vi "Dashboard Main.vi"() -> ()   [LabVIEW 2014]
uses:
  <vilib>/event_ctls.llb/eventvkey.ctl
  <vilib>/Rock Robotics/WPI/Dashboard/WPI_DashboardLogging Global.vi
  <vilib>/Rock Robotics/Network Tables/SD Read Numeric Array.vi
  <vilib>/Rock Robotics/Network Tables/SD Read Number.vi
  <vilib>/Rock Robotics/Network Tables/SD Write Number.vi
  <vilib>/Rock Robotics/Network Tables/SD Read Boolean.vi
  <vilib>/Utility/config.llb/Write Key (String).vi
  <vilib>/Utility/config.llb/Write Key (I32).vi
  <vilib>/Utility/config.llb/NI_LVConfig.lvlib
  <vilib>/Rock Robotics/Network Tables/SD Write String Array.vi
  <vilib>/Rock Robotics/Network Tables/SD Read String Array.vi
panel:
  out "Boolean":bool
  in  "Close Dashboard":bool
  in  "TCP":refnum<k5>
  in  "Rec Mode":enum32{"Stop", "Record", "Playback"}(radio)
  in  "Vision":u16(ring)=3 items=["Camera Off", "USB Camera SW", "USB Camera HW", "IP Camera"]
  out "Image Message":string="Timeout in Camera Communications"
  in  "Dashboard Tab":T1(tab)
  out "Current":dbl[](graph)
  out "Mutton Tank":dbl(knob) scale=0.0..6.0
  in  "AutoMode":enum16{"", "Straight", "Diagonal", "U-Turn"}(ring)
  in  "Camera Settings":T2={"Frame Rate"=30, "Compression"=30, "Size"=1} {"Frame Rate" scale=1.0..30.0; "Size" items=["640x480", "320x240", "160x120"]}
  out "Mode":T3(ring)=enum."Auto Disabled"
  in  "DB Camera Config":bool
  out "fps":dbl format="%#.1g"
  out "Mbps":dbl format="%#.1g"
  out "Mbps 2":bool
  out "Left Pwr":cluster{dbl, dbl}(slide)={0.0, -15.348837209302326} scale=-100.0..100.0
  out "Right Pwr":cluster{dbl, dbl}(slide)={0.0, -15.348837209302326} scale=-100.0..100.0
  out "Right Spd":dbl(slide) scale=-20.0..20.0
  out "Left Spd":dbl(slide) scale=-20.0..20.0
  out "High Gear?":bool
  in  "DB/String 9":string
  in  "DB/String 8":string
  in  "DB/String 7":string
  in  "DB/String 6":string
  in  "DB/String 5":string
  in  "DB/String 4":string
  in  "DB/String 3":string
  in  "DB/String 2":string
  in  "DB/String 1":string
  in  "DB/String 0":string
  in  "DB/Slider 0":dbl(slide) scale=0.0..5.0
  in  "DB/Slider 1":dbl(slide) scale=0.0..5.0
  in  "DB/Slider 2":dbl(slide) scale=0.0..5.0
  in  "DB/Slider 3":dbl(slide) scale=0.0..5.0
  out "DB/LED 3":bool
  out "DB/LED 2":bool
  out "DB/LED 1":bool
  out "DB/LED 0":bool
  in  "DB/Button 3":bool
  in  "DB/Button 2":bool
  in  "DB/Button 1":bool
  in  "DB/Button 0":bool caption="New Name"
  in  "Test Slider":dbl(slide) scale=0.0..100.0 scale format="%#_3g"
  in  "On/Off":bool caption="Solenoid"
  in  "Test Name":u16(ring) items=["Select the test to run...", "Example Test", "-------------------------------", "List of tests is built in robot code.", "Replace with your own automated tests."]
  in  "Test Tree":string(tree)
  in  "Motor":cluster{"Value":dbl, "Enable":bool} {"Value" scale=-1.0..1.0 scale format="%#_3g"}
  out "Progress":T4 {"Test Progress" scale=0.0..100.0}
  in  "Rev/Fwd":cluster{"Forward":bool, "Reverse":bool}
  in  "Test Ring":u16(ring) items=["Monochrome", "Color"]
  in  "Listbox":i32(listbox)
  out "Tree":string(tree)
  in  "Variables":string[](array[string])
  out "Camera Image":T5(plugin-control)
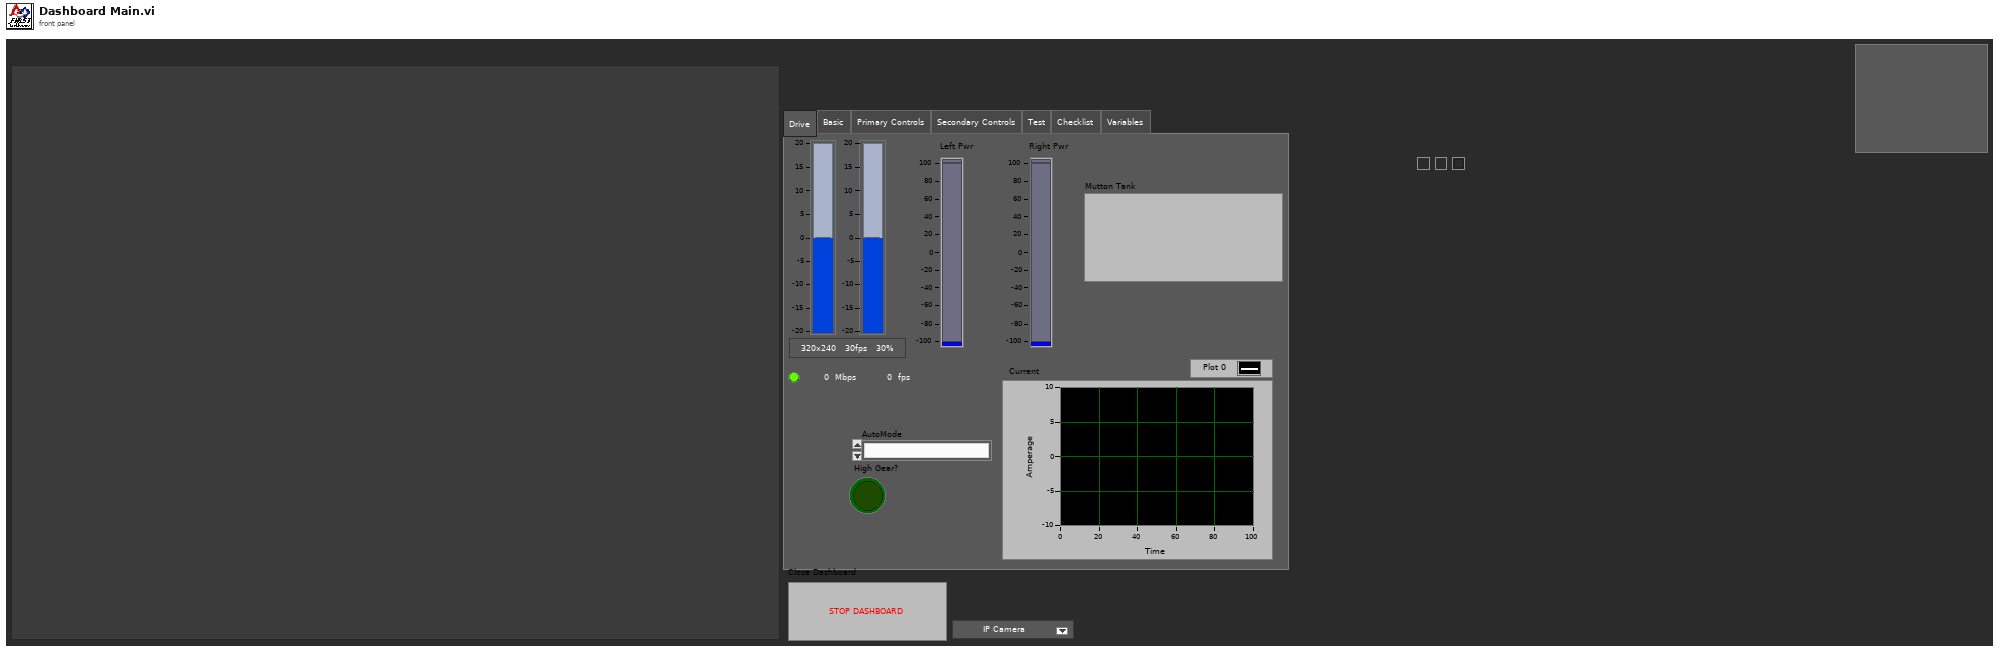
[diagram p1: front panel]
types:
  T1 = enum32{"Drive", "Basic", "Primary Controls", "Secondary Controls", "Test", "Checklist", "Variables"}
  T2 = cluster{"Frame Rate":i32, "Compression":i32, "Size":u16}
  T3 = enum8{"Tele-Op Disabled", "Tele-Op Enabled", "Auto Disabled", "Auto Enabled", "Test Disabled", "Test Enabled", "Disconnected", "No Code", "E-Stop"}
  T4 = cluster{"Test Progress":u8, "Test Progress Text":string}
  T5 = typedef "IMAQ Image.ctl" = refnum<image>
  T6 = enum32{"Drive", "Basic", "Custom", "Test", "Checklist", "Variables"}
  T7 = typedef "Image Type" = u32
  T8 = cluster{"Error Strings":string, "Disable Counts":cluster{u16, u16}, "Rail Faults":cluster{u16, u16, u16}, "Robot IP":string, "DB Mode":u8, "Event Info":cluster{"Name":string, "Type":u8, "Number":u16, "Replay":u8}, "Camera Addr":string}
  T9 = cluster{"Storage":cluster{"Disk Free":u64, "RAM Block":u32, "RAM free":u32}, "CPU Utilization":cluster{"CPU % ISR":sgl, "CPU % Time Crit":sgl, "CPU % Timed Str":sgl, "CPU % High":sgl, "CPU % Above":sgl, "CPU % Normal":sgl, "CPU % Low":sgl}, "CAN":cluster{"% Bus Utilization":sgl, "Bus Off Cnt":u32, "TX_FIFO Full Cnt":u32, "Receive Error Cnt":u8, "Transmit Error Cnt":u8}, "HID":cluster{"HID Outputs":u32, "Rumble Low":u16, "Rumble High":u16}[]}
  T10 = cluster{"Status bits":cluster{"Test Mode":bool, "Autonomous":bool, "Enabled":bool, "Code Start":bool, "Brownout":bool, "Reserved 2":bool, "Reserved 3":bool, "E-Stop":bool}, "Code Trace":cluster{"Disabled":bool, "TeleOp":bool, "Auto":bool, "Test":bool}, "Controller Type":enum16{"unknown", "cRIO", "roboRio"}, "Code?":enum16{"unknown", "noCode", "code"}, "Battery V":dbl}
  T11 = cluster{"Control Bits":cluster{"TestMode":bool, "Autonomous":bool, "Enabled":bool, "FMS Present":bool, bool, bool, bool, "E-Stop":bool}, "Team Station ":u8, "Countdown":sgl, "Joystick Values":cluster{"Axes":dbl[], "Buttons":bool[], "POVs":i16[]}[]}
  T12 = cluster{"Camera Image":refnum<vi>, "Dashboard Tab":refnum<vi>, "Boolean":refnum<vi>, "Vision":refnum<vi>, "Rec Mode":refnum<vi>, "Test Slider":refnum<vi>, "On/Off ":refnum<vi>, "Test Ring":refnum<vi>, "Rev/Fwd":refnum<vi>, "Test Name":refnum<vi>, "Motor":refnum<vi>, "Progress":refnum<vi>, "CheckList":refnum<vi>, "Tree":refnum<vi>, "Test Tree":refnum<vi>}
  T13 = typedef "NI_LVConfig.lvlib/Config Data RefNum.ctl" = refnum<k1>
  T14 = cluster{"Operation":enum16{"Update", "Clear"}, "Color Box":u32}[]
  T15 = typedef "eventvkey.ctl" = enum16{"ASCII", "Enter", "Return", "Shift", "Ctrl", "Alt", "Cmd", "Opt", "Caps", "NumLock", "Clear", "Break", "Up", "Down", "Left", "Right", "Insert", "Delete", "Home", "End", "PageUp", "PageDown", "Escape", "Help", "Pause", "ScrollLock", "F1", "F2", "F3", "F4", "F5", "F6", "F7", "F8", "F9", "F10", "F11", "F12", "F13", "F14", "F15", "F16", "F17", "F18", "F19", "F20", "F21", "F22", "F23", "F24", "Play", "VolumeUp", "VolumeDown", "Mute", "Two Byte Char"}
  T16 = cluster{"Image Size":bool, "Image Type":bool, "Pixel Value":bool, "ROI Information":bool, "Zoom Factor":bool}
  T17 = enum8{"Enabled", "Disabled", "Disabled and Grayed Out"}
  T18 = cluster{"Operation":enum16{"Update", "Clear"}, "Color Box":u32}
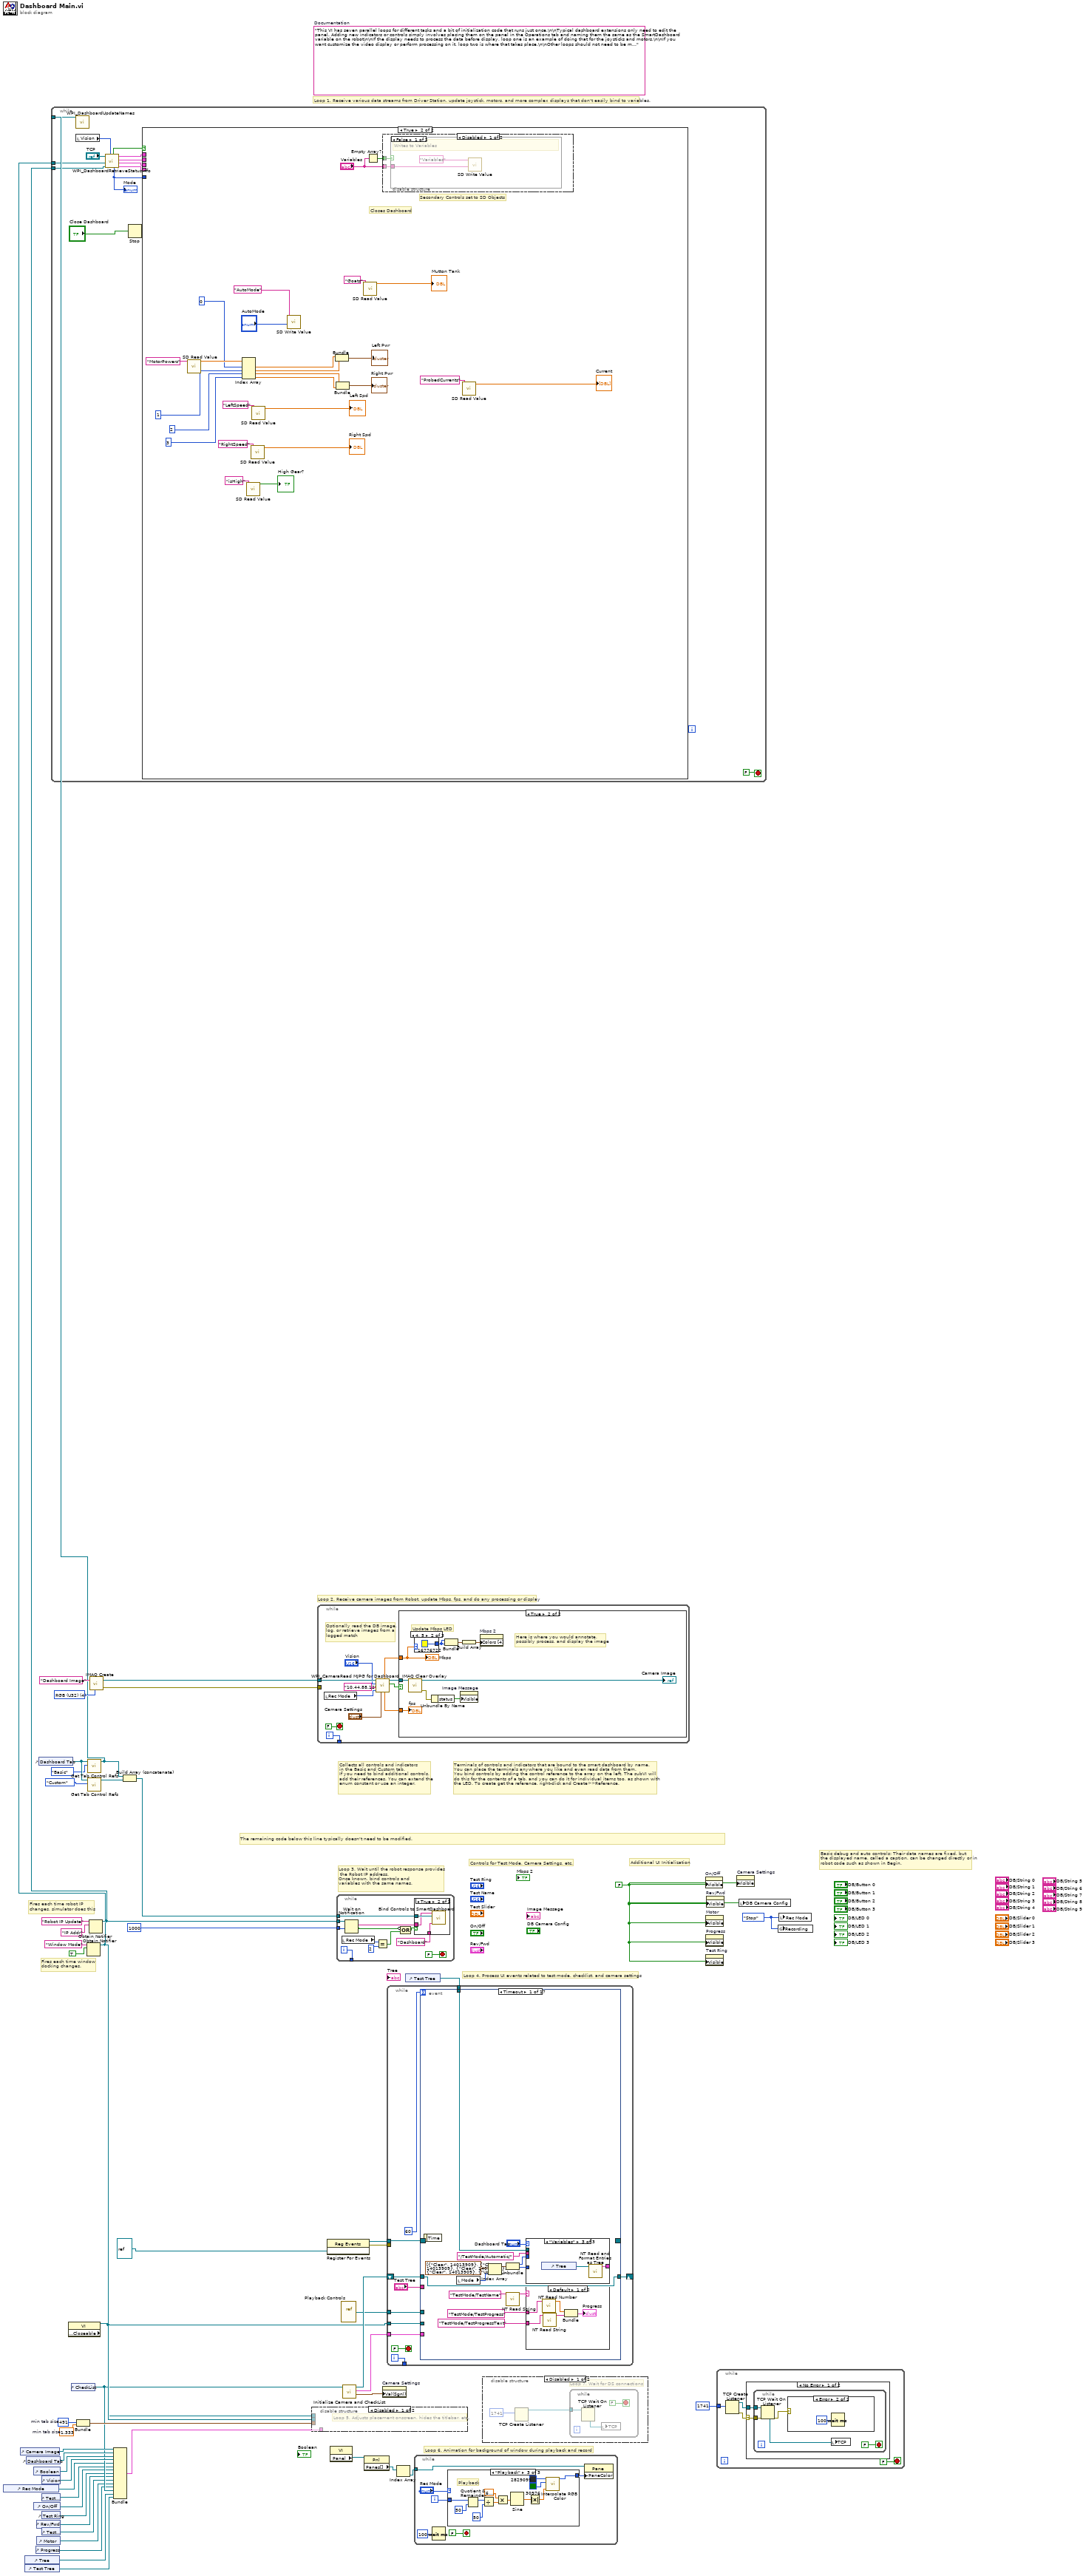
[diagram p0: block diagram]
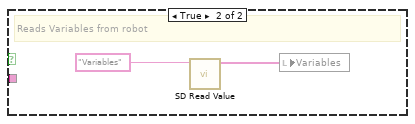
[diagram p7: hidden frame]
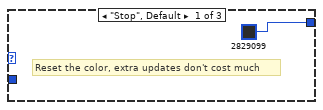
[diagram p9: hidden frame]
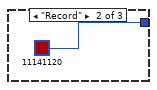
[diagram p10: hidden frame]
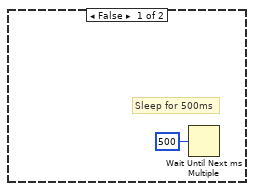
[diagram p12: hidden frame]
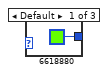
[diagram p13: hidden frame]
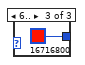
[diagram p14: hidden frame]
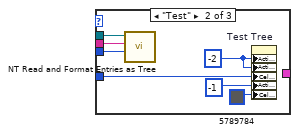
[diagram p16: hidden frame]
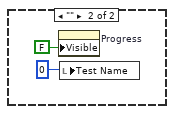
[diagram p17: hidden frame]
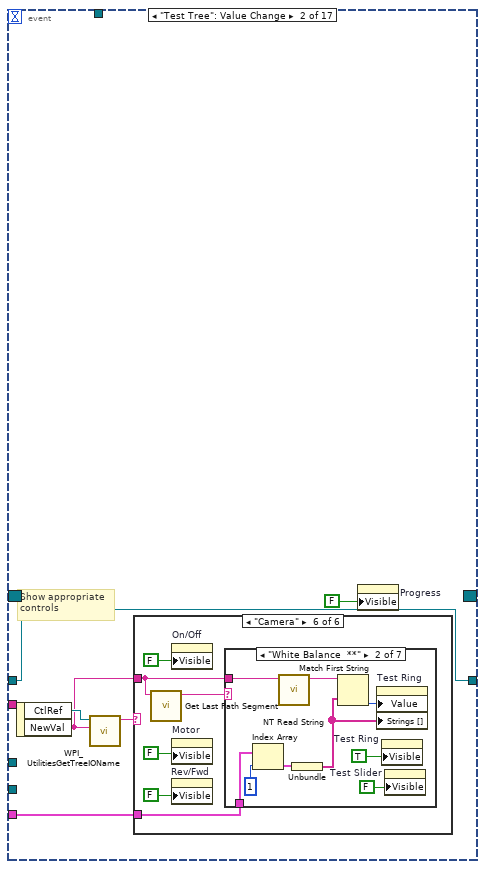
[diagram p18: hidden frame]
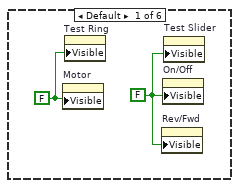
[diagram p19: hidden frame]
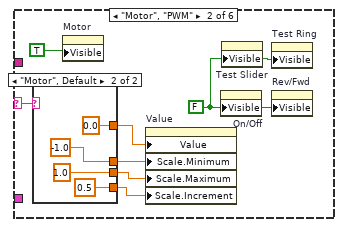
[diagram p20: hidden frame]
diagram:
  w23 = 491  # min tab size
  w22 = 1.333  # min tab size
  w31 = enum32{"Stop", "Record", "Playback"}."Stop" ("Rec Mode")
  w5 = FALSE ("Visible")
  (unwired) "This VI has seven parallel loops for different tasks and a bit of initialization code that runs just once.\n\nTypical dashboard extensions only need to edit the panel. Adding new indicators or controls simply involves placing them on the panel in the Operations tab and naming them the same as the SmartDashboard variable on the robot\n\nIf the display needs to process the data before display, loop one is an example of doing that for the joysticks and motors.\n\nIf you want customize the video display or perform processing on it, loop two is where that takes place.\n\nOther loops should not need to be modified. They are pretty standard, and document the task they perform."  # Documentation
  w51 = T7 4 items=["Grayscale (U8)", "Grayscale (I16)", "Grayscale (SGL)", "Complex (CSG)", "RGB (U32)", "HSL (U32)", "RGB (U64)"] ("Image Type")
  # "Basic debug and auto controls: Their data names are fixed, but\nthe displayed name, called a caption, can be changed directly or in\nrobot code such as shown in Begin."
  # "Controls for Test Mode, Camera Settings, etc."
  # "Additional UI Initialization"
  # "Loop 6. Animation for background of window during playback and record"
  # "Fires each time robot IP\nchanges, simulator does this"
  # "Fires each time window\ndocking changes."
  # "Collects all controls and indicators\nin the Basic and Custom tab.\nIf you need to bind additional controls,\nadd their references. You can extend the\nenum constant or use an integer."
  # "The remaining code below this line typically doesn't need to be modified."
  # "Loop 4. Process UI events related to test mode, checklist, and camera settings"
  # "Terminals of controls and indicators that are bound to the smart dashboard by name.\nYou can place the terminals anywhere you like and even read data from them.\nYou bind controls by adding the control reference to the array on the left. The subVI will\ndo this for the contents of a tab, and you can do it for individual items too, as shown with\nthe LED. To create get the reference, right-click and Create>>Reference."
  # "Loop 3. Wait until the robot response provides\n the Robot IP address.\nOnce known, bind controls and\nvariables with the same names."
  # "Loop 1. Receive various data streams from Driver Station, update joystick, motors, and more complex displays that don't easily bind to variables."
  # "Loop 2. Receive camera images from Robot, update Mbps, fps, and do any processing or display"
  n1 = control-ref of="Rec Mode"() -> (w11:refnum<vi>)
  n2 = control-ref of="Camera Image"() -> (w26:refnum<vi>)
  n3 = control-ref of="Tree"() -> (w15:refnum<vi>)
  n4 = control-ref of="Test Tree"() -> (w14:refnum<vi>)
  n5 = control-ref of="Dashboard Tab"() -> (w25:refnum<vi>)
  n6 = control-ref of="Boolean"() -> (w20:refnum<vi>)
  n7 = control-ref of="On/Off"() -> (w9:refnum<vi>)
  n8 = control-ref of="Progress"() -> (w6:refnum<vi>)
  n9 = control-ref of="Rev/Fwd"() -> (w7:refnum<vi>)
  n10 = control-ref of="Motor"() -> (w12:refnum<vi>)
  n11 = control-ref of="Dashboard Tab"() -> (w29:refnum<vi>)
  n12 = control-ref of="Test Slider"() -> (w10:refnum<vi>)
  n13 = control-ref of="Vision"() -> (w24:refnum<vi>)
  n14 = control-ref of="Test Ring"() -> (w8:refnum<vi>)
  n15 = control-ref of="Test Name"() -> (w13:refnum<vi>)
  n16 = property class="VI" props=["Front Panel.Closeable"]() -> (reference out=w30:refnum<vi>)  [unwired: 2 in, 2 out]
  n17 = control-ref of="CheckList"() -> (w16:refnum<vi>)
  n18 = Bundle("min tab size"=w23, "min tab size"=w22) -> (w21:cluster{"min tab size":i32, "min tab size":dbl})  [unwired: 1 in]
  n19 = Obtain Notifier(name (unnamed)="Window Mode", notification data type=TRUE) -> (notifier out=w2:refnum<notifier>)  [unwired: 2 in, 2 out]
  n20 = call <vilib>:"Get Tab Control Refs.vi"("Page Index"=T6."Basic" ("Dashboard Tab"), "TabControl in"=w29) -> ("ControlsOnPage"=w3:refnum<vi>[])  [unwired: 9 in]
  n21 = call <vilib>:"Get Tab Control Refs.vi"("Page Index"=T6."Custom" ("Dashboard Tab"), "TabControl in"=w29) -> ("ControlsOnPage"=w28:refnum<vi>[])  [unwired: 9 in]
  n22 = Obtain Notifier(name (unnamed)="Robot IP Update", notification data type="IP Addr" ("name (unnamed)")) -> (notifier out=w4:refnum<notifier>)  [unwired: 2 in, 2 out]
  n23 = while {
    tunnel: w4 -> [w59]
    tunnel: w3 -> [w58]
    tunnel: w2 -> [w54]
    stop <- FALSE stop-if-true
    n24 = call <vilib>:"WPI_DashboardUpdateNames.vi"("Controls on Tab"=w58) -> ()  [unwired: 11 in]
    n25 = local read "Vision"() -> (w56:u16)
    n26 = call <vilib>:"WPI_DashboardRetrieveStatusInfo.vi"("Vision"=w56, "Binding Refnum"=w59, "Window Mode Notifier"=w54, "TCP Cnx"="TCP") -> ("Power and Errors"=w60:T8, "Robot Metrics"=w63:T9, "Status Info"=w64:T10, "Control Info"=w61:T11, "Robot Mode"=w57:T3, "Process?"=w62:bool)  [unwired: 2 in]
    "Mode" <- w57
    n27 = Stop(stop? (T)="Close Dashboard") -> ()
    n28 = case shown="True" w62 {
      tunnel: w64 -> [_ _]
      tunnel: w63 -> [_ _]
      tunnel: w61 -> [_ _]
      tunnel: w60 -> [_ _]
      tunnel: w57 -> [_ _]
      frame False {
      }
      frame True {
        # "Closes Dashboard"
        # "Secondary Controls set to SD Objects"
        n29 = call-poly <vilib>:"SD Read Value.vi"("Name"="MotorPowers") -> ("Numeric Array"=w87:dbl[])  [unwired: 8 in, 2 out]
        n30 = Index Array(array=w87, index #1=0 ("index"), index #2=1 ("index"), index #3=2 ("index"), index #4=3 ("index")) -> (element #1=w77:dbl, element #2=w76:dbl, element #3=w74:dbl, element #4=w73:dbl)
        n31 = call-poly <vilib>:"SD Read Value.vi"("Name"="isHigh") -> ("Boolean"=→"High Gear?":bool)  [unwired: 8 in, 2 out]
        n32 = call-poly <vilib>:"SD Read Value.vi"("Name"="RightSpeed") -> ("Numeric"=→"Right Spd":dbl)  [unwired: 8 in, 2 out]
        n33 = call-poly <vilib>:"SD Read Value.vi"("Name"="LeftSpeed") -> ("Numeric"=→"Left Spd":dbl)  [unwired: 8 in, 2 out]
        n34 = call-poly <vilib>:"SD Write Value.vi"("Numeric"="AutoMode", "Name"="AutoMode") -> ()  [unwired: 8 in, 2 out]
        n35 = Bundle("Numeric"=w77, "Numeric"=w76) -> (→"Left Pwr":cluster{"Numeric":dbl, "Numeric":dbl})  [unwired: 1 in]
        n36 = Bundle("Numeric"=w74, "Numeric"=w73) -> (→"Right Pwr":cluster{"Numeric":dbl, "Numeric":dbl})  [unwired: 1 in]
        n37 = call-poly <vilib>:"SD Read Value.vi"("Name"="Goats") -> ("Numeric"=→"Mutton Tank":dbl)  [unwired: 8 in, 2 out]
        n38 = Empty Array?(array="Variables") -> (empty?=w90:bool)
        n39 = disable-structure shown="Disabled" {
          disable-tunnel: w90 -> [w92 _]
          disable-tunnel: "Variables" -> [w91 _]
          frame Disabled {
            n40 = case shown="False" w92 {
              tunnel: w91 -> [w93 _]
              frame False {
                # "Writes to Variables"
                n41 = call-poly <vilib>:"SD Write Value.vi"("String Array"=w93, "Name"="Variables") -> ()  [unwired: 8 in, 2 out]
              }
              frame True {
                # "Reads Variables from robot"
                n42 = call-poly <vilib>:"SD Read Value.vi"("Name"="Variables") -> ("String Array"=w95:string[])  [unwired: 9 in, 1 out]
                n43 = local write "Variables"(w95) -> ()
              }
            }
          }
          frame Enabled {
          }
        }
        n44 = call-poly <vilib>:"SD Read Value.vi"("Name"="ProbedCurrents") -> ("Numeric Array"=→"Current":dbl[])  [unwired: 8 in, 2 out]
      }
    }
  }
  n45 = call "IMAQ Create"("Image Name"="Dashboard Image", "Image Type"=w51) -> ("New Image"=w49:T5, "error out"=w48:errorcluster)  [unwired: 2 in, 1 out]
  n46 = Bundle("Camera Image"=w26, "Dashboard Tab"=w25, "Boolean"=w20, "Vision"=w24, "Rec Mode"=w11, "Test Slider"=w10, "On/Off"=w9, "Test Ring"=w8, "Rev/Fwd"=w7, "Test Name"=w13, "Motor"=w12, "Progress"=w6, "CheckList"=w16, "Tree"=w15, "Test Tree"=w14) -> (w17:T12)  [unwired: 1 in]
  n47 = Build Array (concatenate)(w3, w28) -> (w27:refnum<vi>[])
  n48 = disable-structure shown="Disabled" {
    disable-tunnel: w30 -> [_ _]
    disable-tunnel: w21 -> [_ _]
    disable-tunnel: w17 -> [_ _]
    disable-tunnel: w2 -> [_ _]
    frame Disabled {
      # "Loop 5. Adjusts placement onscreen, hides the titlebar, etc."
    }
    frame Enabled {
    }
  }
  n49 = while {
    tunnel: w49 -> [w105]
    tunnel: w48 -> [_]
    tunnel: [w106] -> _
    i -> [w106]
    stop <- FALSE stop-if-true
    # "Optionally read the DB image,\nlog, or retrieve images from a\nlogged match"
    n50 = local read "Rec Mode"() -> (w99:enum32{"Stop", "Record", "Playback"})
    n51 = call <vilib>:"WPI_CameraRead MJPG for Dashboard.vi"("Camera Settings"="Camera Settings", "Rec Mode"=w99, "Camera IP"="10.44.88.12", "Camera Mode"="Vision", "Refnum in"=w105) -> ("Active"=w103:bool, "Refnum out"=w104:T5, "FPS"=w102:dbl, "Bandwidth (Mbps)"=w101:dbl)  [unwired: 3 in]
    n52 = case shown="True" w103 {
      tunnel: w104 -> [_ w112]
      tunnel: w101 -> [_ w111]
      tunnel: w102 -> [_ w109]
      frame False {
        # "Sleep for 500ms"
        n53 = Wait Until Next ms Multiple(millisecond multiple=u32 500) -> ()  [unwired: 1 out]
      }
      frame True {
        # "Here is where you would annotate,\npossibly process, and display the image"
        # "Update Mbps LED"
        n54 = call "IMAQ Clear Overlay"("Image"=w112) -> ("error out"=w116:errorcluster, "Image Out"=→"Camera Image":T5)  [unwired: 2 in, 7 out]
        n55 = case shown="4, 5" w111 {
          tunnel: [u32 6618880 ("Color Box") u32 16776722 ("Color Box") u32 16716800 ("Color Box")] -> w113
          frame Default {
          }
          frame 4, 5 {
          }
          frame 6.. {
          }
        }
        n56 = Unbundle By Name(w116) -> ("status"=w117:bool)
        n57 = Bundle("Color Box"=w113, "Color Box"=w113) -> (w115:cluster{"Color Box":u32, "Color Box":u32})  [unwired: 1 out]
        n58 = property on="Image Message" class="Str"("Visible"=w117) -> ()  [unwired: 2 in, 2 out]
        n59 = Build Array(w115) -> (w114:cluster{"Color Box":u32, "Color Box":u32}[])
        n60 = property on="Mbps 2" class="Bool (strict)"("Colors [4]"=w114) -> ()  [unwired: 2 in, 2 out]
        "Mbps" <- w111
        "fps" <- w109
      }
    }
  }
  n61 = register-events(refnum<vi> refnum) -> (reference out=w35:refnum<event-registration>, error out=w34:errorcluster)  [unwired: 2 in]
  n62 = property class="VI"() -> ("Panel"=w38:refnum<vi>)  [unwired: 2 in, 2 out]
  n63 = while {
    tunnel: w27 -> [w132]
    tunnel: w4 -> [w130]
    tunnel: [w128] -> _
    tunnel: u32 1000 ("milliseconds to wait") -> [w127]
    i -> [w128]
    stop <- FALSE stop-if-true
    n64 = local read "Rec Mode"() -> (w123:enum32{"Stop", "Record", "Playback"})
    n65 = Wait on Notification(notifier=w130, timeout in ms (-1)=w127) -> (notification=w129:string, timed out?=w125:bool)  [unwired: 2 in, 2 out]
    n66 = Equal?(x=w123, y=u16 2 ("Rec Mode")) -> (x = y?=w124:bool)
    n67 = Compound Arithmetic op=OR(invert w125, w124) -> (w126:bool)
    n68 = case shown="True" w126 {
      tunnel: w132 -> [_ w135]
      tunnel: w129 -> [_ w134]
      tunnel: "Dashboard" -> [_ w133]
      frame False {
      }
      frame True {
        n69 = call <vilib>:"Bind Controls to SmartDashboard.vi"("Client Name"=w133, "Bound Control Refs"=w135, "Server IP Address"=w134) -> ()  [unwired: 9 in]
      }
    }
  }
  n70 = vi-ref "Playback Controls.vi"() -> (w36:refnum<vi>)
  n71 = call "Initialize Camera and CheckList.vi"("ListBox in"=w16) -> ("Cluster"=w42:cluster{"value":i32, "value":i32, "index":i32}, "Array"=w43:cluster{string[]}[], "File Refnum"=w41:T13)  [unwired: 8 in]
  n72 = property class="Pnl"(reference=w38) -> ("Panes[]"=w39:refnum<vi>[])  [unwired: 1 in, 2 out]
  n73 = property on="Camera Settings" class="Clust (strict)"("Val(Sgnl)"=w42) -> ()  [unwired: 2 in, 2 out]
  n74 = Index Array(array=w39) -> (element=w37:refnum<vi>)  [unwired: 1 in]
  n75 = control-ref of="Test Tree"() -> (w40:refnum<vi>)
  n76 = while {
    tunnel: w43 -> [w143]
    shift-right: [w142] -> _
    shift-left: w41 -> [w141]
    tunnel: [w140] -> _
    tunnel: w40 -> [w139]
    tunnel: w36 -> [w138]
    tunnel: w35 -> [w137]
    tunnel: w34 -> [_]
    tunnel: w30 -> [w136]
    i -> [w140]
    stop <- FALSE stop-if-true
    n77 = event shown="[0] Timeout" {
      selector: w137 -> [_ _ _ _ _ _ _ _ _ _ _ _ _ _ _ _ _]
      dyn-events: [_ _ _ _ _ _ _ _ _ _ _ _ _ w381 _ _ _] -> _
      timeout: u32 60 ("milliseconds to wait") -> [_ _ _ _ _ _ _ _ _ _ _ _ _ _ _ _ _]
      tunnel: w139 -> [w155 _ _ _ _ _ _ _ _ _ _ _ _ _ _ _ _]
      tunnel: "Test Tree" -> [_ _ _ _ _ _ _ _ w350 w358 w360 w364 w372 _ _ _ _]
      tunnel: w143 -> [_ w177 _ _ _ _ w314 w344 _ _ _ _ _ _ _ _ _]
      tunnel: [w151 w176 w275 w280 w288 w300 w313 w337 w349 w356 w359 w363 w371 w383 w397 w398 w408] -> w142
      tunnel: w141 -> [w151 w176 w275 w280 w288 w300 w312 w337 w349 w356 w359 w363 w371 w383 w397 w398 w408]
      tunnel: w138 -> [_ _ _ _ _ _ _ _ _ _ _ _ _ w384 _ w401 _]
      tunnel: w136 -> [_ _ _ _ _ _ _ _ _ _ _ _ _ w379 _ _ _]
      event Timeout {
        n78 = event-data() -> ()  [unwired: 1 in, 1 out]
        n79 = local read "Mode"() -> (w154:T3)
        n80 = Index Array(array=T14 [{"Operation"=enum."Clear", "Color Box"=14013909}, {"Operation"=enum."Clear", "Color Box"=14013909}, {"Operation"=enum."Clear", "Color Box"=14013909}, {"Operation"=enum."Clear", "Color Box"=14013909}, {"Operation"=enum."Update", "Color Box"=14013909}, {"Operation"=enum."Update", "Color Box"=16777215}, {"Operation"=enum."Clear", "Color Box"=14013909}, {"Operation"=enum."Clear", "Color Box"=14013909}, {"Operation"=enum."Clear", "Color Box"=14013909}], index=w154) -> (element=w149:T18)
        n81 = Unbundle(w149) -> ("Operation"=w148:enum16{"Update", "Clear"}, "Color Box"=w147:u32)
        n82 = call <vilib>:"NT Read String.vi"("Name"="TestMode/TestName") -> ("String"=w158:string)  [unwired: 9 in, 1 out]
        n83 = case shown="\"Variables\"" "Dashboard Tab" {
          tunnel: w155 -> [_ w166 _]
          tunnel: "/TestMode/Automatic/" ("Name Pattern") -> [_ w165 _]
          tunnel: w148 -> [_ w164 _]
          tunnel: [_ _ w168] -> _
          tunnel: w147 -> [_ w160 _]
          frame "Primary Controls", Default {
          }
          frame "Test" {
            w163 = -2 ("Active Item:Row Number")
            n84 = call <vilib>:"NT Read and Format Entries as Tree.vi"("Operation"=w164, "Name Pattern"=w165, "Tree Refnum"=w166) -> ()  [unwired: 7 in, 2 out]
            n85 = property on="Test Tree" class="Tree (strict)"("Active Item Row Number"=w163, "ActiveColNum"=w163, "CellBG"=w160, "Active Item Row Number"=-1 ("Active Item:Row Number"), "CellBG"=u32 5789784 ("Color Box")) -> ()  [unwired: 2 in, 2 out]
          }
          frame "Variables" {
            n86 = control-ref of="Tree"() -> (w167:refnum<vi>)
            n87 = call <vilib>:"NT Read and Format Entries as Tree.vi"("Tree Refnum"=w167) -> ("Formatted Strings"=w168:cluster{"Name":string, "Value":string}[])  [unwired: 9 in, 1 out]
          }
        }
        n88 = case shown="Default" w158 {
          tunnel: "TestMode/TestProgress" ("Name") -> [w170 _]
          tunnel: "TestMode/TestProgressText" ("Name") -> [w169 _]
          frame Default {
            n89 = call <vilib>:"NT Read Number.vi"("Name"=w170) -> ("Numeric"=w171:dbl)  [unwired: 9 in, 1 out]
            n90 = call <vilib>:"NT Read String.vi"("Name"=w169) -> ("String"=w172:string)  [unwired: 9 in, 1 out]
            n91 = Bundle("Numeric"=w171, "String"=w172) -> (→"Progress":cluster{"Numeric":dbl, "String":string})  [unwired: 1 in]
          }
          frame "" {
            n92 = property on="Progress" class="Clust (strict)"("Visible"=FALSE) -> ()  [unwired: 2 in, 2 out]
            n93 = local write "Test Name"(u16 0) -> ()
          }
        }
      }
      event "Test Tree": Value Change {
        # "Show appropriate\ncontrols"
        n94 = event-data() -> ("CtlRef"=w180:refnum<vi>, "NewVal"=w178:string)  [unwired: 1 in]
        n95 = call <vilib>:"WPI_UtilitiesGetTreeIOName.vi"("NewVal"=w178, "TreeControl in"=w180) -> ("I/O Name"=w181:string)  [unwired: 9 in]
        n96 = case shown="\"Camera\"" w181 {
          selector: w181 -> [_ w188 _ w206 w215 _]
          tunnel: w178 -> [_ _ w203 w205 _ w222]
          tunnel: w177 -> [_ _ _ _ _ w221]
          frame Default {
            w183 = FALSE ("Visible")
            w182 = FALSE ("Visible")
            n97 = property on="Motor" class="Clust (strict)"("Visible"=w182) -> ()  [unwired: 2 in, 2 out]
            n98 = property on="Test Ring" class="Ring (strict)"("Visible"=w182) -> ()  [unwired: 2 in, 2 out]
            n99 = property on="Rev/Fwd" class="Clust (strict)"("Visible"=w183) -> ()  [unwired: 2 in, 2 out]
            n100 = property on="On/Off" class="Bool (strict)"("Visible"=w183) -> ()  [unwired: 2 in, 2 out]
            n101 = property on="Test Slider" class="Slide (strict)"("Visible"=w183) -> ()  [unwired: 2 in, 2 out]
          }
          frame "Motor", "PWM" {
            w189 = FALSE ("Visible")
            n102 = case shown="\"Motor\", Default" w188 {
              tunnel: [1.0 ("Value") -1.0 ("Value")] -> w187
              tunnel: [255.0 ("Value") 1.0 ("Value")] -> w186
              tunnel: [128.0 ("Value") 0.0 ("Value")] -> w185
              tunnel: [64.0 ("Value") 0.5 ("Value")] -> w184
              frame "PWM" {
              }
              frame "Motor", Default {
              }
            }
            n103 = property on="Motor" class="Clust (strict)"("Visible"=TRUE) -> ()  [unwired: 2 in, 2 out]
            n104 = property on="Value" class="Slide (strict)"("Value"=w185, "Scale.Minimum"=w187, "Scale.Maximum"=w186, "Scale.Increment"=w184) -> ()  [unwired: 2 in, 2 out]
            n105 = property on="On/Off" class="Bool (strict)"("Visible"=w189) -> ()  [unwired: 2 in, 2 out]
            n106 = property on="Test Slider" class="Slide (strict)"("Visible"=w189) -> ()  [unwired: 2 in, 2 out]
            n107 = property on="Test Ring" class="Ring (strict)"("Visible"=w189) -> ()  [unwired: 2 in, 2 out]
            n108 = property on="Rev/Fwd" class="Clust (strict)"("Visible"=w189) -> ()  [unwired: 2 in, 2 out]
          }
          frame "Servo" {
            w201 = FALSE ("Visible")
            n109 = call <vilib>:"NT Read Number.vi"("Name"=w203) -> ("Numeric"=w202:dbl)  [unwired: 9 in, 1 out]
            n110 = property on="Test Slider" class="Slide (strict)"("Visible"=TRUE, "Scale.Maximum"=170.0 ("Scale.Range:Maximum")) -> ()  [unwired: 2 in, 2 out]
            n111 = local write "Test Slider"(w202) -> ()
            n112 = property on="Motor" class="Clust (strict)"("Visible"=w201) -> ()  [unwired: 2 in, 2 out]
            n113 = property on="Rev/Fwd" class="Clust (strict)"("Visible"=w201) -> ()  [unwired: 2 in, 2 out]
            n114 = property on="On/Off" class="Bool (strict)"("Visible"=w201) -> ()  [unwired: 2 in, 2 out]
            n115 = property on="Test Ring" class="Ring (strict)"("Visible"=w201) -> ()  [unwired: 2 in, 2 out]
          }
          frame "Relay", "Solenoid" {
            w204 = FALSE ("Visible")
            n116 = property on="Motor" class="Clust (strict)"("Visible"=w204) -> ()  [unwired: 2 in, 2 out]
            n117 = property on="Test Slider" class="Slide (strict)"("Visible"=w204) -> ()  [unwired: 2 in, 2 out]
            n118 = Search and Replace String(input string=w205, search string="/Value  **", replace string="/Direction") -> (result string=w211:string)  [unwired: 5 in, 3 out]
            n119 = property on="Test Ring" class="Ring (strict)"("Visible"=w204) -> ()  [unwired: 2 in, 2 out]
            n120 = call <vilib>:"NT Read String.vi"("Name"=w211) -> ("String"=w209:string)  [unwired: 9 in, 1 out]
            n121 = Equal?(x="Both directions", y=w209) -> (x = y?=w207:bool)
            n122 = Not(x=w207) -> (.not. x?=w208:bool)
            n123 = property on="Rev/Fwd" class="Clust (strict)"("Visible"=w207) -> ()  [unwired: 2 in, 2 out]
            n124 = property on="On/Off" class="Bool (strict)"("Visible"=w208, "Caption.Text"=w206) -> ()  [unwired: 2 in, 2 out]
          }
          frame "Compressor", "Digital Out" {
            w214 = FALSE ("Visible")
            # "Get direction and finish"
            n125 = property on="Motor" class="Clust (strict)"("Visible"=w214) -> ()  [unwired: 2 in, 2 out]
            n126 = property on="Test Slider" class="Slide (strict)"("Visible"=w214) -> ()  [unwired: 2 in, 2 out]
            n127 = property on="Test Ring" class="Ring (strict)"("Visible"=w214) -> ()  [unwired: 2 in, 2 out]
            n128 = property on="On/Off" class="Bool (strict)"("Visible"=TRUE, "Caption.Text"=w215) -> ()  [unwired: 2 in, 2 out]
            n129 = property on="Rev/Fwd" class="Clust (strict)"("Visible"=FALSE) -> ()  [unwired: 2 in, 2 out]
          }
          frame "Camera" {
            n130 = call <vilib>:"Get Last Path Segment.vi"("String in"=w222) -> ("String out"=w223:string)  [unwired: 10 in]
            n131 = property on="On/Off" class="Bool (strict)"("Visible"=FALSE) -> ()  [unwired: 2 in, 2 out]
            n132 = property on="Motor" class="Clust (strict)"("Visible"=FALSE) -> ()  [unwired: 2 in, 2 out]
            n133 = property on="Rev/Fwd" class="Clust (strict)"("Visible"=FALSE) -> ()  [unwired: 2 in, 2 out]
            n134 = case shown="\"White Balance  **\"" w223 {
              tunnel: w222 -> [w229 w238 w247 w256 w265 _ w271]
              tunnel: w221 -> [w227 w235 w244 w253 w262 _ _]
              frame "Size  **" {
                n135 = Index Array(array=w227) -> (element=w226:cluster{string[]})  [unwired: 1 in]
                n136 = call <vilib>:"NT Read String.vi"("Name"=w229) -> ("String"=w228:string)  [unwired: 9 in, 1 out]
                n137 = Unbundle(w226) -> (w224:string[])
                n138 = Match First String(2:w224, 3:w228) -> (0:w225:i32)  [unwired: 1 out]
                n139 = property on="Test Ring" class="Ring (strict)"("Value"=w225, "Strings []"=w224) -> ()  [unwired: 2 in, 2 out]
                n140 = property on="Test Ring" class="Ring (strict)"("Visible"=TRUE) -> ()  [unwired: 2 in, 2 out]
                n141 = property on="Test Slider" class="Slide (strict)"("Visible"=FALSE) -> ()  [unwired: 2 in, 2 out]
              }
              frame "White Balance  **" {
                n142 = Index Array(array=w235, index=1) -> (element=w236:cluster{string[]})
                n143 = call <vilib>:"NT Read String.vi"("Name"=w238) -> ("String"=w237:string)  [unwired: 9 in, 1 out]
                n144 = Unbundle(w236) -> (w233:string[])
                n145 = Match First String(2:w233, 3:w237) -> (0:w232:i32)  [unwired: 1 out]
                n146 = property on="Test Ring" class="Ring (strict)"("Value"=w232, "Strings []"=w233) -> ()  [unwired: 2 in, 2 out]
                n147 = property on="Test Ring" class="Ring (strict)"("Visible"=TRUE) -> ()  [unwired: 2 in, 2 out]
                n148 = property on="Test Slider" class="Slide (strict)"("Visible"=FALSE) -> ()  [unwired: 2 in, 2 out]
              }
              frame "Exposure  **" {
                n149 = Index Array(array=w244, index=2) -> (element=w245:cluster{string[]})
                n150 = call <vilib>:"NT Read String.vi"("Name"=w247) -> ("String"=w246:string)  [unwired: 9 in, 1 out]
                n151 = Unbundle(w245) -> (w241:string[])
                n152 = Match First String(2:w241, 3:w246) -> (0:w242:i32)  [unwired: 1 out]
                n153 = property on="Test Ring" class="Ring (strict)"("Value"=w242, "Strings []"=w241) -> ()  [unwired: 2 in, 2 out]
                n154 = property on="Test Ring" class="Ring (strict)"("Visible"=TRUE) -> ()  [unwired: 2 in, 2 out]
                n155 = property on="Test Slider" class="Slide (strict)"("Visible"=FALSE) -> ()  [unwired: 2 in, 2 out]
              }
              frame "Exposure Priority  **" {
                n156 = Index Array(array=w253, index=3) -> (element=w254:cluster{string[]})
                n157 = call <vilib>:"NT Read String.vi"("Name"=w256) -> ("String"=w255:string)  [unwired: 9 in, 1 out]
                n158 = Unbundle(w254) -> (w250:string[])
                n159 = Match First String(2:w250, 3:w255) -> (0:w251:i32)  [unwired: 1 out]
                n160 = property on="Test Ring" class="Ring (strict)"("Value"=w251, "Strings []"=w250) -> ()  [unwired: 2 in, 2 out]
                n161 = property on="Test Ring" class="Ring (strict)"("Visible"=TRUE) -> ()  [unwired: 2 in, 2 out]
                n162 = property on="Test Slider" class="Slide (strict)"("Visible"=FALSE) -> ()  [unwired: 2 in, 2 out]
              }
              frame "Color Enable  **" {
                n163 = Index Array(array=w262, index=4) -> (element=w263:cluster{string[]})
                n164 = call <vilib>:"NT Read String.vi"("Name"=w265) -> ("String"=w264:string)  [unwired: 9 in, 1 out]
                n165 = Unbundle(w263) -> (w259:string[])
                n166 = Match First String(2:w259, 3:w264) -> (0:w260:i32)  [unwired: 1 out]
                n167 = property on="Test Ring" class="Ring (strict)"("Value"=w260, "Strings []"=w259) -> ()  [unwired: 2 in, 2 out]
                n168 = property on="Test Ring" class="Ring (strict)"("Visible"=TRUE) -> ()  [unwired: 2 in, 2 out]
                n169 = property on="Test Slider" class="Slide (strict)"("Visible"=FALSE) -> ()  [unwired: 2 in, 2 out]
              }
              frame Default {
                n170 = property on="Test Ring" class="Ring (strict)"("Visible"=FALSE) -> ()  [unwired: 2 in, 2 out]
                n171 = property on="Test Slider" class="Slide (strict)"("Visible"=FALSE) -> ()  [unwired: 2 in, 2 out]
              }
              frame "Brightness  **", "Color Level  **", "Compression  **", "FPS  **", "Sharpness  **" {
                n172 = call <vilib>:"NT Read Number.vi"("Name"=w271) -> ("Numeric"=w270:dbl)  [unwired: 9 in, 1 out]
                n173 = local write "Test Slider"(w270) -> ()
                n174 = property on="Test Slider" class="Slide (strict)"("Visible"=TRUE, "Scale.Maximum"=100.0 ("Scale.Range:Maximum")) -> ()  [unwired: 2 in, 2 out]
                n175 = property on="Test Ring" class="Ring (strict)"("Visible"=FALSE) -> ()  [unwired: 2 in, 2 out]
              }
            }
          }
        }
        n176 = property on="Progress" class="Clust (strict)"("Visible"=FALSE) -> ()  [unwired: 2 in, 2 out]
      }
      event "Test Name": Mouse Enter {
        # "Populate the ring with the list of tests"
        n177 = event-data() -> ()  [unwired: 1 in, 1 out]
        n178 = call <vilib>:"NT Read String Array.vi"("Name"="TestMode/TestList") -> ("String Array"=w279:string[])  [unwired: 9 in, 1 out]
        n179 = Build Array (concatenate)("Select the test to run...", w279) -> (w278:string[])
        n180 = property on="Test Name" class="Ring (strict)"("Strings []"=w278) -> ()  [unwired: 2 in, 2 out]
      }
      event "Test Name": Value Change {
        w281 = FALSE ("Visible")
        # "Tell the robot the test name to run"
        n181 = event-data() -> ("NewVal"=w285:u16)  [unwired: 1 in]
        n182 = property on="Test Name" class="Ring (strict)"() -> ("Strings []"=w286:string[])  [unwired: 2 in, 2 out]
        n183 = local write "Progress"(T4 {"Test Progress"=0, "Test Progress Text"=""} ("Progress")) -> ()
        n184 = Index Array(array=w286, index=w285) -> (element=w284:string)
        n185 = call <vilib>:"NT Write String.vi"("String"=w284, "Name"="TestMode/TestName") -> ()  [unwired: 9 in, 1 out]
        n186 = property on="Progress" class="Clust (strict)"("Visible"=TRUE) -> ()  [unwired: 2 in, 2 out]
        n187 = property on="Motor" class="Clust (strict)"("Visible"=w281) -> ()  [unwired: 2 in, 2 out]
        n188 = property on="Test Slider" class="Slide (strict)"("Visible"=w281) -> ()  [unwired: 2 in, 2 out]
        n189 = property on="On/Off" class="Bool (strict)"("Visible"=w281) -> ()  [unwired: 2 in, 2 out]
        n190 = property on="Rev/Fwd" class="Clust (strict)"("Visible"=w281) -> ()  [unwired: 2 in, 2 out]
        n191 = property on="Test Ring" class="Ring (strict)"("Visible"=w281) -> ()  [unwired: 2 in, 2 out]
      }
      event "Listbox": Double Click {
        # "Shift clears all"
        # "Update symbols on the listbox"
        n192 = event-data() -> ("PlatMods.Shift"=w289:bool, "Row"=w291:i32)  [unwired: 1 in]
        n193 = case shown="True" w289 {
          tunnel: w291 -> [w295 _]
          tunnel: 1 -> [w294 _]
          frame False {
            n194 = property on="Listbox" class="LstBox (strict)"() -> ("Item Symbols"=w293:i32[])  [unwired: 2 in, 2 out]
            n195 = Replace Array Subset(array=w293, new element=w294, index=w295) -> (w292:i32[])
            n196 = property on="Listbox" class="LstBox (strict)"("Item Symbols"=w292) -> ()  [unwired: 2 in, 2 out]
          }
          frame True {
            w296 = 0 ("Top Row")
            n197 = property on="Listbox" class="LstBox (strict)"() -> ("Number of Rows"=w298:u32)  [unwired: 2 in, 2 out]
            n198 = Initialize Array(0, w298) -> (w297:i32[])
            n199 = property on="Listbox" class="LstBox (strict)"("Top Row"=w296, "Value"=w296, "Item Symbols"=w297) -> ()  [unwired: 2 in, 2 out]
          }
        }
      }
      event "Listbox": Key Down {
        # "Update symbols on the listbox\nLeft and right keys check and uncheck"
        n200 = event-data() -> ("VKey"=w302:T15)  [unwired: 1 in]
        n201 = case shown="\"Left\", \"Right\"" w302 {
          selector: w302 -> [w307 _]
          tunnel: eventvkey."Left" ("VKey") -> [w305 _]
          frame "Left", "Right" {
            n202 = Equal?(x=w305, y=w307) -> (x = y?=w306:bool)
            n203 = Select(t=0, s=w306, f=1) -> (s? t:f=w308:i32)
            n204 = property on="Listbox" class="LstBox (strict)"() -> ("Item Symbols"=w311:i32[])  [unwired: 2 in, 2 out]
            n205 = Replace Array Subset(array=w311, new element=w308, index="Listbox") -> (w310:i32[])
            n206 = property on="Listbox" class="LstBox (strict)"("Item Symbols"=w310) -> ()  [unwired: 2 in, 2 out]
          }
          frame Default {
          }
        }
      }
      event "DB Camera Config": Value Change {
        # "Show or hide the cluster of controls, store in ini file"
        n207 = event-data() -> ("NewVal"=w315:bool)  [unwired: 1 in]
        n208 = case shown="False" w315 {
          tunnel: w314 -> [w324 _]
          tunnel: [w317 w335] -> w313
          tunnel: w312 -> [w316 w335]
          frame False {
            w331 = "Camera"
            w334 = FALSE ("Visible")
            n209 = local read "Camera Settings"() -> (w323:T2)
            n210 = Index Array(array=w324) -> (element=w327:cluster{string[]})  [unwired: 1 in]
            n211 = Unbundle(w323) -> ("Frame Rate"=w322:i32, "Compression"=w321:i32, "Size"=w325:u16)
            n212 = Unbundle(w327) -> (w326:string[])
            n213 = Index Array(array=w326, index=w325) -> (element=w320:string)
            n214 = call-poly <vilib>:"Write Key.vi"("section"=w331, "value"=w320, "key"="Size", "refnum"=w316) -> ("refnum out"=w333:T13)  [unwired: 2 in, 5 out]
            n215 = call-poly <vilib>:"Write Key.vi"("section"=w331, "value"=w322, "key"="FrameRate", "refnum"=w333) -> ("refnum out"=w332:T13)  [unwired: 1 in, 6 out]
            n216 = property on="Camera Settings" class="Clust (strict)"("Visible"=w334) -> ()  [unwired: 2 in, 2 out]
            n217 = local write "DB Camera Config"(w334) -> ()
            n218 = call-poly <vilib>:"Write Key.vi"("section"=w331, "value"=w321, "key"="Compression", "refnum"=w332) -> ("refnum out"=w318:T13)  [unwired: 1 in, 6 out]
            n219 = call <vilib>:"Close Config Data.vi"("refnum"=w318) -> ("file path"=w319:path)  [unwired: 2 in, 8 out]
            n220 = call <vilib>:"Open Config Data.vi"("configuration file path"=w319) -> ("refnum"=w317:T13)  [unwired: 8 in, 2 out]
          }
          frame True {
            n221 = property on="Camera Settings" class="Clust (strict)"("Visible"=TRUE) -> ()  [unwired: 2 in, 2 out]
          }
        }
      }
      event "Camera Settings": Value Change {
        # "Update summary string when any elements of DB camera change"
        n222 = event-data() -> ("NewVal"=w348:T2)  [unwired: 1 in]
        n223 = Index Array(array=w344) -> (element=w343:cluster{string[]})  [unwired: 1 in]
        n224 = Unbundle(w348) -> ("Frame Rate"=w339:i32, "Compression"=w338:i32, "Size"=w341:u16)
        n225 = Unbundle(w343) -> (w342:string[])
        n226 = Index Array(array=w342, index=w341) -> (element=w340:string)
        n227 = Format Into String(format string="%s   %dfps   %d%%", w340, w339, w338) -> (resulting string=w345:string)  [unwired: 2 in, 1 out]
        n228 = Build Array(w345) -> (w346:string[])
        n229 = property on="DB Camera Config" class="Bool (strict)"("Strings [4]"=w346) -> ()  [unwired: 2 in, 2 out]
      }
      event "Motor.Enable": Value Change {
        # "When the test mode otor enable helper is set, update that\ntree row item's value"
        n230 = event-data() -> ("NewVal"=w354:bool)  [unwired: 1 in]
        n231 = Unbundle("Motor") -> ("Value"=w353:dbl)  [unwired: 1 out]
        n232 = Select(t=w353, s=w354, f=0.0) -> (s? t:f=w351:dbl)
        n233 = call <vilib>:"NT Write Number.vi"("Numeric"=w351, "Name"=w350) -> ()  [unwired: 9 in, 1 out]
      }
      event "Test Slider": Value Change {
        # "When the test mode slider helper is set, update that\ntree row item's value"
        n234 = event-data() -> ("NewVal"=w357:dbl)  [unwired: 1 in]
        n235 = call <vilib>:"NT Write Number.vi"("Numeric"=w357, "Name"=w358) -> ()  [unwired: 9 in, 1 out]
      }
      event "On/Off": Value Change {
        # "When the test mode on/off helper value is set, update that\ntree row item's value"
        n236 = event-data() -> ("NewVal"=w362:bool)  [unwired: 1 in]
        n237 = Boolean To (0,1)(Boolean=w362) -> (0, 1=w361:i16)
        n238 = call <vilib>:"NT Write Number.vi"("Numeric"=w361, "Name"=w360) -> ()  [unwired: 9 in, 1 out]
      }
      event "Rev/Fwd": Value Change {
        # "When the test mode helper value for relays is set, update that\ntree row item's value"
        n239 = event-data() -> ("NewVal.Forward"=w370:bool, "NewVal.Reverse"=w369:bool)  [unwired: 1 in]
        n240 = Boolean To (0,1)(Boolean=w370) -> (0, 1=w366:i16)
        n241 = Boolean To (0,1)(Boolean=w369) -> (0, 1=w368:i16)
        n242 = Negate(x=w368) -> (-x=w367:i16)
        n243 = Add(x=w366, y=w367) -> (x+y=w365:i16)
        n244 = call <vilib>:"NT Write Number.vi"("Numeric"=w365, "Name"=w364) -> ()  [unwired: 9 in, 1 out]
      }
      event "Test Ring": Value Change {
        # "When a test mode helper value is selected from the ring,\nset the tree item's variable to the string value"
        n245 = event-data() -> ("NewVal"=w374:u16)  [unwired: 1 in]
        n246 = property on="Test Ring" class="Ring (strict)"() -> ("Strings []"=w375:string[])  [unwired: 2 in, 2 out]
        n247 = Index Array(array=w375, index=w374) -> (element=w373:string)
        n248 = call <vilib>:"NT Write String.vi"("String"=w373, "Name"=w372) -> ()  [unwired: 9 in, 1 out]
      }
      event "Rec Mode": Value Change {
        # "Update globals for recording mode and path to read log from.\nClear when logging and let NetworkTables set path for vision to\nuse."
        n249 = event-data() -> ("NewVal"=w385:enum32{"Stop", "Record", "Playback"})  [unwired: 1 in]
        n250 = global write "WPI_DashboardLogging Global.vi" "Logging Filename"(path "") -> ()
        n251 = case shown="\"Playback\"" w385 {
          tunnel: w384 -> [_ w387 w395]
          tunnel: [_ _ w394] -> w381
          tunnel: [_ _ w393] -> _
          tunnel: w379 -> [_ _ w391]
          tunnel: cluster{i32, i32} {-250, 170} -> [_ _ w390]
          tunnel: [_ _ T16 {"Image Size"=TRUE, "Image Type"=TRUE, "Pixel Value"=TRUE, "ROI Information"=TRUE, "Zoom Factor"=FALSE} ("Image Information Shown:All Elements")] -> w377
          tunnel: [_ _ TRUE ("Zoom Factor")] -> w376
          frame Default {
          }
          frame "Stop", "Record" {
            # "Place Window too"
            n252 = invoke class="VI" method="FP.Close"(reference=w387) -> (reference out=w386:refnum<vi>)  [unwired: 2 in, 2 out]
            n253 = invoke class="VI" method="Abort VI"(reference=w386) -> ()  [unwired: 2 in, 3 out]
          }
          frame "Playback" {
            n254 = call "Open Playback Panel.vi"("Offset"=w390, "DB VI Ref"=w391, "Playback in"=w395) -> ("Playback out"=w392:refnum<vi>)  [unwired: 8 in]
            n255 = register-events(w392) -> (reference out=w394:refnum<event-registration>, error out=w393:errorcluster)  [unwired: 2 in]
          }
        }
        n256 = global write "WPI_DashboardLogging Global.vi" "Recording"(w385) -> ()
        n257 = property on="Camera Image" class="ImageControl"("Image Information Shown"=w377, "Image Information Visible"=w376) -> ()  [unwired: 2 in, 2 out]
        n258 = call <vilib>:"WPI_DashboardNT Log FieldName Cache.vi"("Operation"=enum16{"Lookup/Add", "Index", "Clear"}."Clear") -> ()  [unwired: 8 in, 3 out]
      }
      event Panel Close {
        w396 = enum32{"Stop", "Record", "Playback"}."Stop" ("Rec Mode")
        # "Playback window has been closed, abort"
        n259 = event-data() -> ()  [unwired: 1 in, 4 out]
        n260 = local write "Rec Mode"(w396) -> ()
        n261 = global write "WPI_DashboardLogging Global.vi" "Recording"(w396) -> ()
      }
      event Panel Close {
        # "Abort playback window and ourself"
        n262 = event-data() -> ()  [unwired: 1 in, 4 out]
        n263 = invoke class="VI" method="FP.Close"(reference=w401) -> (reference out=w400:refnum<vi>)  [unwired: 2 in, 2 out]
        n264 = invoke class="VI" method="Abort VI"(reference=w400) -> (error out=w399:errorcluster)  [unwired: 2 in, 2 out]
        n265 = invoke class="VI" method="Abort VI"(error in=w399) -> ()  [unwired: 2 in, 3 out]
      }
      event "Vision": Value Change {
        # "Enable/Disable Compression slider.\nHW USB is hard-coded into the camera"
        n266 = event-data() -> ("NewVal"=w407:u16)  [unwired: 1 in]
        n267 = Equal?(x=w407, y=u32 2 ("milliseconds to wait")) -> (x = y?=w405:bool)
        n268 = Select(t=T17."Disabled and Grayed Out" ("Disabled"), s=w405, f=T17."Enabled" ("Disabled")) -> (s? t:f=w402:T17)
        n269 = property on="Compression" class="Slide (strict)"("DisabledEnum"=w402) -> ()  [unwired: 2 in, 2 out]
      }
    }
  }
  n270 = while {
    tunnel: w37 -> [w410]
    i -> [w413]
    stop <- FALSE stop-if-true
    n271 = Wait (ms)(milliseconds to wait=u32 100) -> ()  [unwired: 1 out]
    n272 = case shown="\"Playback\"" "Rec Mode" {
      tunnel: w413 -> [_ _ w428]
      tunnel: [u32 2829099 ("Base Color") u32 11141120 ("Target Color") w417] -> w409
      frame "Stop", Default {
        # "Reset the color, extra updates don't cost much"
      }
      frame "Record" {
      }
      frame "Playback" {
        # "Playback"
        n273 = Quotient & Remainder(x=w428, y=u32 50 ("milliseconds to wait")) -> (x-y*floor(x/y)=w424:u32)  [unwired: 1 out]
        n274 = Divide(x=w424, y=u32 50 ("milliseconds to wait")) -> (x/y=w421:dbl)
        n275 = Multiply(x=6.283185307179586, y=w421) -> (x*y=w426:dbl)
        n276 = Sine(x=w426) -> (sin(x)=w425:dbl)
        n277 = Absolute Value(x=w425) -> (abs(x)=w418:dbl)
        n278 = call "Interpolate RGB Color.vi"("Proportion"=w418, "Target Color"=u32 30976, "Base Color"=u32 2829099) -> ("Result Color"=w417:u32)  [unwired: 8 in]
      }
    }
    n279 = property class="Pane"(reference=w410, "PaneColor"=w409) -> ()  [unwired: 1 in, 2 out]
  }
  n280 = disable-structure shown="Disabled" {
    frame Disabled {
      # "Loop 7. Wait for DS connections"
      n281 = TCP Create Listener(10:u16 1741 ("timeout ms (25000)")) -> (3:w429:refnum<k5>)  [unwired: 4 in, 2 out]
      n282 = while {
        tunnel: w429 -> [w432]
        stop <- FALSE stop-if-true
        n283 = TCP Wait On Listener(11:w432) -> (4:w431:refnum<k5>)  [unwired: 3 in, 4 out]
        n284 = local write "TCP"(w431) -> ()
      }
    }
    frame Enabled {
    }
  }
  n285 = property on="On/Off" class="Bool (strict)"("Visible"=w5) -> ()  [unwired: 2 in, 2 out]
  n286 = property on="Motor" class="Clust (strict)"("Visible"=w5) -> ()  [unwired: 2 in, 2 out]
  n287 = property on="Progress" class="Clust (strict)"("Visible"=w5) -> ()  [unwired: 2 in, 2 out]
  n288 = property on="Test Ring" class="Ring (strict)"("Visible"=w5) -> ()  [unwired: 2 in, 2 out]
  n289 = property on="Rev/Fwd" class="Clust (strict)"("Visible"=w5) -> ()  [unwired: 2 in, 2 out]
  n290 = while {
    tunnel: u16 1741 ("timeout ms (25000)") -> [w437]
    stop <- FALSE stop-if-true
    n291 = TCP Create Listener(10:w437) -> (0:w436:errorcluster, 3:w434:refnum<k5>)  [unwired: 4 in, 1 out]
    n292 = case shown="No Error" w436 {
      selector: w436 -> [w439 _]
      tunnel: w434 -> [w438 _]
      frame No Error {
        n293 = while {
          tunnel: w439 -> [w443]
          tunnel: w438 -> [w440]
          stop <- FALSE stop-if-true
          n294 = TCP Wait On Listener(8:w443, 11:w440) -> (0:w442:errorcluster, 4:w441:refnum<k5>)  [unwired: 2 in, 3 out]
          n295 = case shown="Error" w442 {
            frame No Error {
            }
            frame Error {
              n296 = Wait (ms)(milliseconds to wait=u32 100) -> ()  [unwired: 1 out]
            }
          }
          n297 = local write "TCP"(w441) -> ()
        }
      }
      frame Error {
      }
    }
  }
  n298 = property on="Camera Settings" class="Clust (strict)"("Visible"=w5) -> ()  [unwired: 2 in, 2 out]
  n299 = local write "DB Camera Config"(w5) -> ()
  n300 = global write "WPI_DashboardLogging Global.vi" "Recording"(w31) -> ()
  n301 = local write "Rec Mode"(w31) -> ()
